vi "Destroy.vi"(8 "error in":errorcluster, 11 "Sorted Object Dictionary in":refnum<class "Sorted Object Dictionary.lvclass">) -> (0 "error out":errorcluster, 3 "Sorted Object Dictionary out":refnum<class "Sorted Object Dictionary.lvclass">)   [LabVIEW 2024, in "EDS.lvlib" / "Sorted Object Dictionary.lvclass"]
uses:
  Sorted Object Dictionary.lvclass
  Sorted Object Dictionary.lvclass/Sorted Object Dictionary.ctl
  OD Entry/OD Entry.lvclass
  OD Sub-Entry/OD Sub-Entry.lvclass
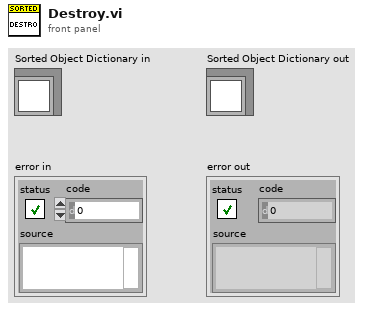
[diagram p1: front panel]
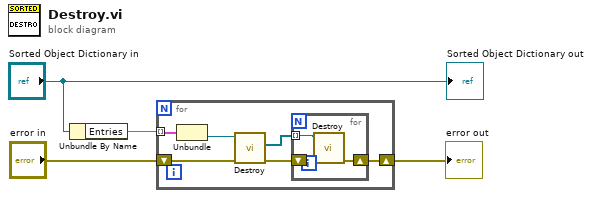
[diagram p0: block diagram]
diagram:
  n1 = Unbundle By Name("Sorted Object Dictionary in") -> ("Entries"=w3:map{u16, refnum<class "OD Entry.lvclass">})
  n2 = for {
    tunnel: w3 -> [w10] mode=indexing
    shift-right: [w6] -> w1
    shift-left: "error in" -> [w8]
    n3 = Unbundle(w10) -> ("OD Entry"=w9:refnum<class "OD Entry.lvclass">)  [unwired: 1 out]
    n4 = call-dynamic "Destroy.vi"("Error In"=w8, "reference in"=w9) -> ("Error Out"=w7:errorcluster, "Sub-Entries"=w5:refnum<class "OD Sub-Entry.lvclass">[])  [unwired: 7 in, 1 out]
    n5 = for {
      shift-right: [w12] -> w6
      shift-left: w7 -> [w13]
      tunnel: w5 -> [w11] mode=indexing
      n6 = call-dynamic "Destroy.vi"("Error In"=w13, "reference in"=w11) -> ("Error Out"=w12:errorcluster)  [unwired: 7 in, 2 out]
    }
  }
  "error out" <- w1
  "Sorted Object Dictionary out" <- "Sorted Object Dictionary in"
